vi "Read Process Variable.vi"(4 "error in (no error)":errorcluster, 7 "Instance Name":T1) -> (0 "error out":errorcluster, 2 "Last Sample Time":dbl[unit], 3 "Last value":dbl)   [LabVIEW 2015, in "Startup Processes.lvlib"]
uses:
  Startup Processes.lvlib
  _typedefs/Subpanel Names.ctl
  <vilib>/ptbypt/NI_PtbyPt.lvlib
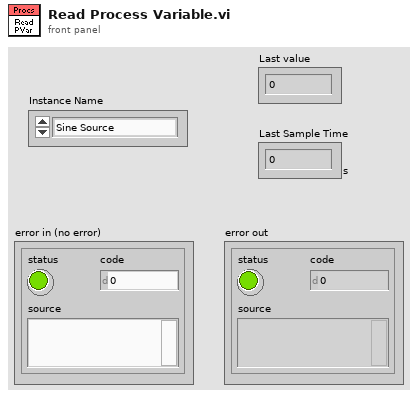
[diagram p1: front panel]
types:
  T1 = typedef "Startup Processes.lvlib/Subpanel Names.ctl" = enum16{"Sine Source", "Ramp Source", "Hen House TC", "Dog House TC", "Out House TC"}
  T2 = enum16{"Write Fan State", "Write Cooler State", "Read"}
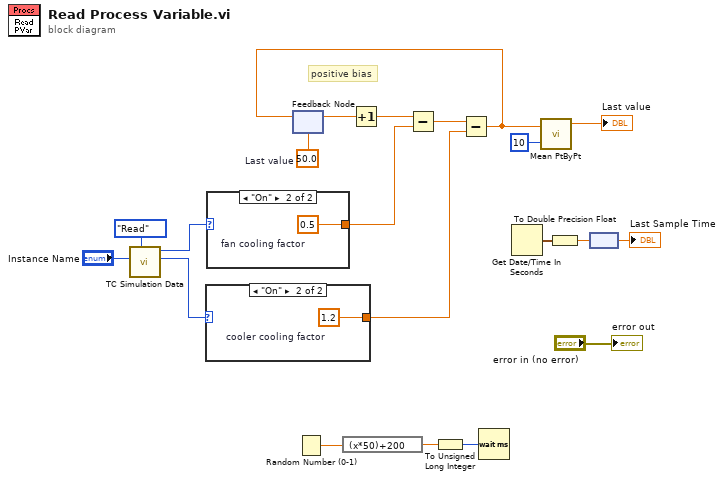
[diagram p0: block diagram]
diagram:
  w19 = 50.0  # Last value
  # "positive bias"
  n1 = call "TC Simulation Data.vi"("Function"=T2."Read", "Machine Name"="Instance Name") -> ("Cooler State"=w11:enum16{"Off", "On"}, "Fan State"=w14:enum16{"Off", "On"})  [unwired: 4 in, 1 out]
  n2 = case shown="\"On\"" w11 {
    tunnel: [_ w21] -> w12
    frame "Off" {
    }
    frame "On" {
      w21 = 1.2  # cooler cooling factor
    }
  }
  n3 = case shown="\"On\"" w14 {
    tunnel: [_ w22] -> w13
    frame "Off" {
    }
    frame "On" {
      w22 = 0.5  # fan cooling factor
    }
  }
  n4 = feedback #1(w19) -> (w18:dbl)
  n5 = Random Number (0-1)() -> (number: 0 to 1=w4:dbl)
  n6 = expression code="(x*50)+200"(w4) -> (w3:dbl)
  n7 = Increment(x=w18) -> (x+1=w16:dbl)
  n8 = Subtract(x=w16, y=w13) -> (x-y=w17:dbl)
  n9 = To Unsigned Long Integer(number=w3) -> (unsigned 32bit integer=w2:u32)
  n10 = Subtract(x=w17, y=w12) -> (x-y=w10:dbl)
  n11 = feedback-in #1(w10) -> ()
  n12 = Wait (ms)(milliseconds to wait=w2) -> ()  [unwired: 1 out]
  n13 = Get Date/Time In Seconds() -> (seconds since 1Jan1904=w7:timestamp)
  n14 = call <vilib>:"Mean PtByPt.vi"("x"=w10, "sample length"=10) -> ("mean"=→"Last value":dbl)  [unwired: 2 in, 1 out]
  n15 = To Double Precision Float(number=w7) -> (double precision float=w6:dbl)
  n16 = node(w6) -> (→"Last Sample Time":dbl[unit])
  "error out" <- "error in (no error)"
